vi "Sprinklernew.vi"() -> ()   [LabVIEW 2013]
doc: "This VI is the simulation of sprinkler controller.\nOn pressing Run the vi will read the data from Logdata.txt file and write it into the Zone Setup Array.\nSetup: On pressing it Zone Setup Array will enable and Zone selector allow the user to select and change the zone:\n-North\n-East\n-South\n-West\nThe controller could handle zones in any order and more than once in Zone Setup Array.\n\n In run selector toggle switch :\n-Single(off): The controller will service the Zone as setup in the zone.\n-Contineous(on):The controller will continue th ecyale as setup in zone till the Stop button will not pressed.\nStart button: It start the controller."
uses:
  Controls/Sprinkler State.ctl
  Controls/Log data states.ctl
panel:
  in  "Setup":bool
  in  "Zone Setup Array":cluster{"Zone Selector":string, "Timing":dbl}[](array[cluster])
  out "Controller Status":string
  out "Zone Indicators":T1
  in  "Water Pressure Sensor (%)":u32(slide) scale=0.0..100.0
  in  "Rain Sensor":bool
  in  "Run Selector":bool
  in  "Start":bool
  in  "stop":bool
  # "Controls"
  # "Simulation Controls"
  # "Rain"
  # "No Rain"
  # "Continuous"
  # "Single"
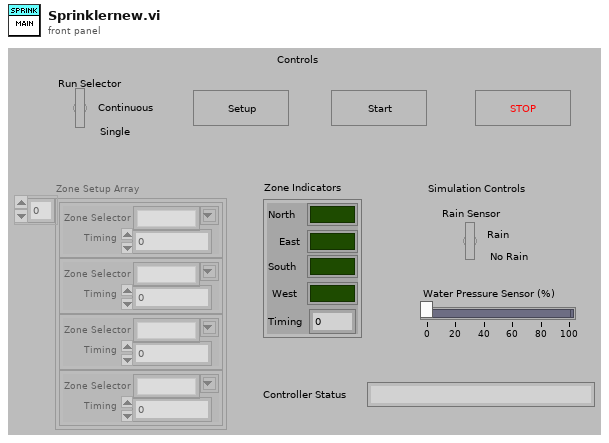
[diagram p1: front panel]
types:
  T1 = cluster{"North":bool, "East":bool, "South":bool, "West":bool, "Timing":u32}
  T2 = typedef "Sprinkler State.ctl" = enum16{"Initialize", "Setup", "Enable Zone", "Select", "Main", "Run Complete", "Rain", "Stop"}
  T3 = typedef "Log data states.ctl" = enum16{"Initialize", "Read", "Write", "Stop"}
  T4 = enum8{"Enabled", "Disabled", "Disabled and Grayed Out"}
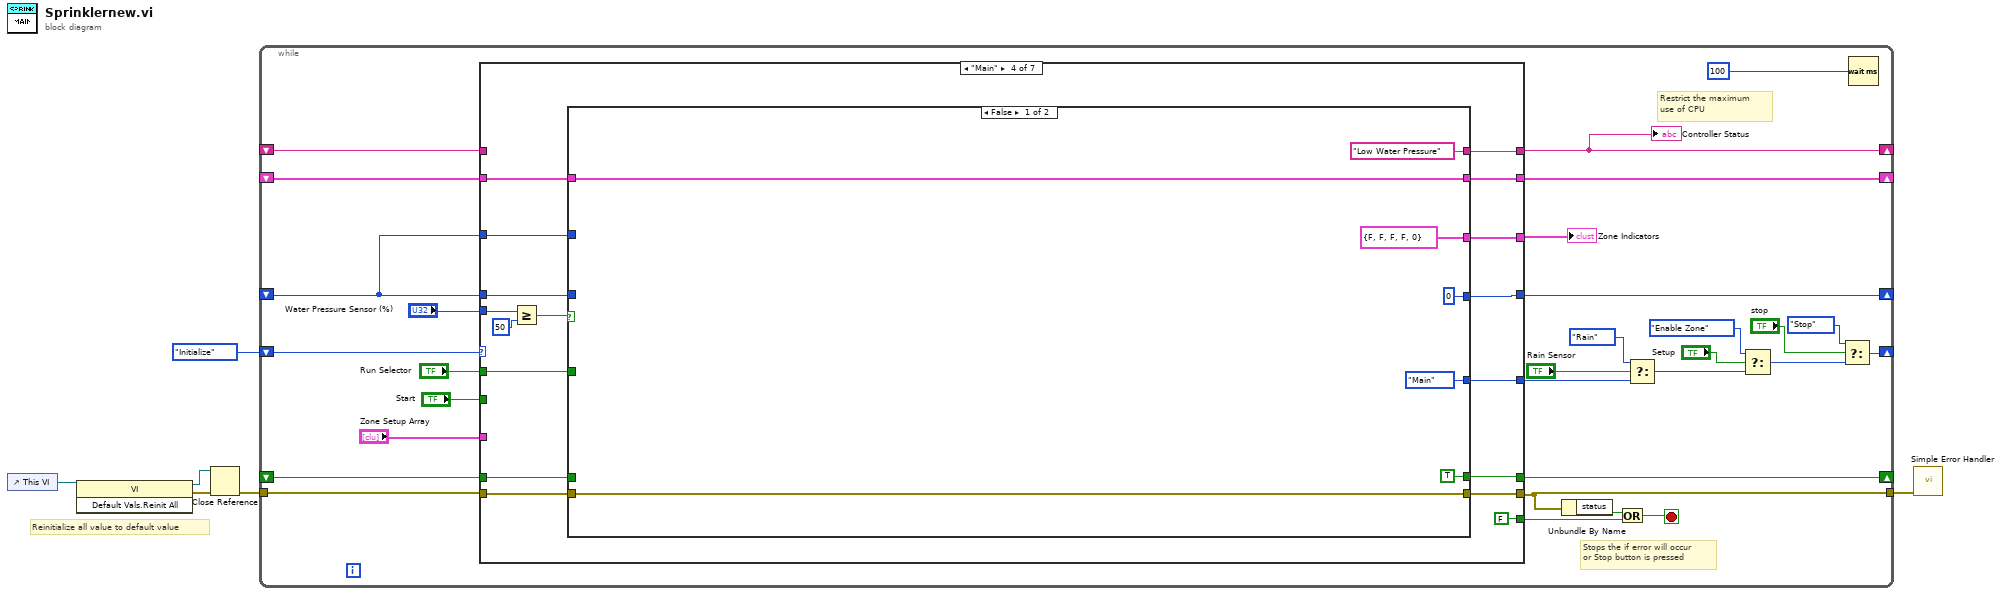
[diagram p0: block diagram]
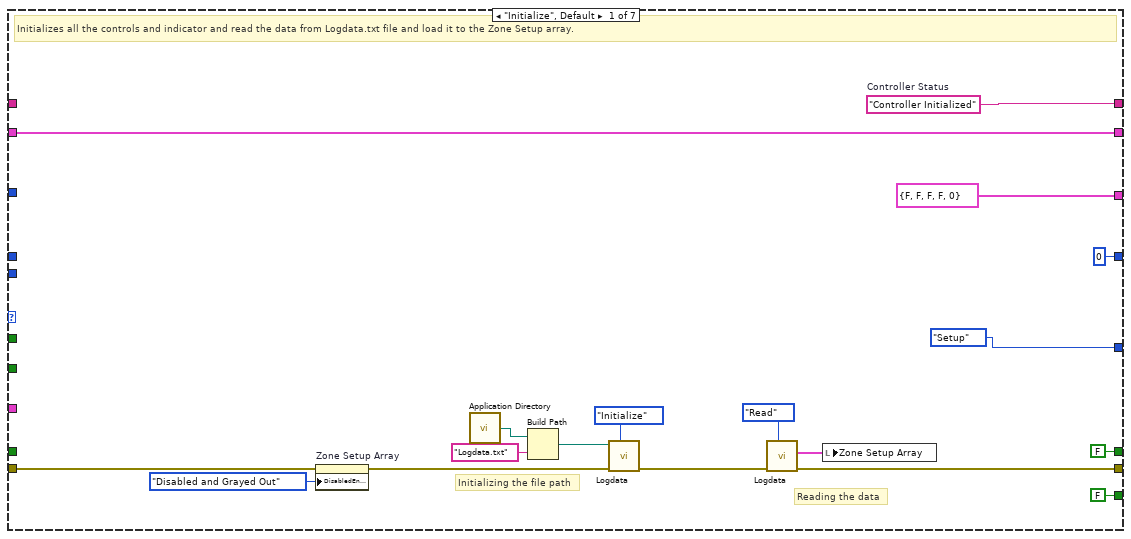
[diagram p2: hidden frame]
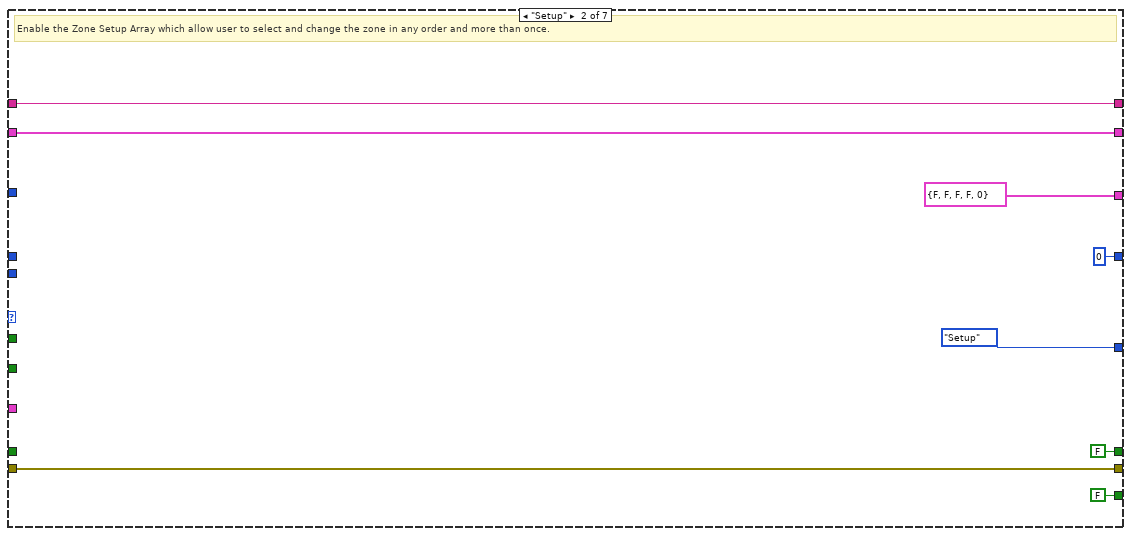
[diagram p3: hidden frame]
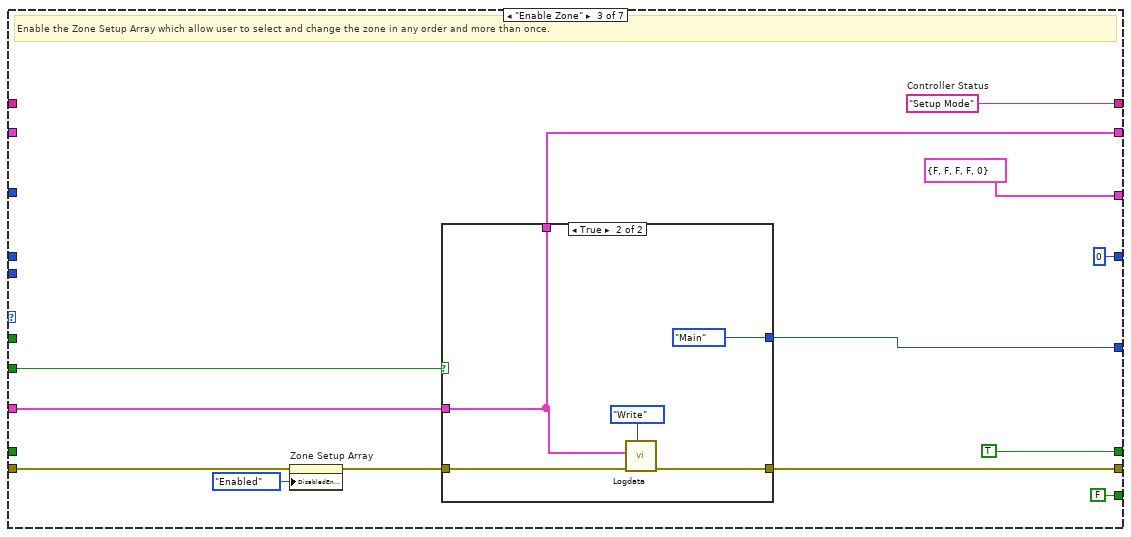
[diagram p4: hidden frame]
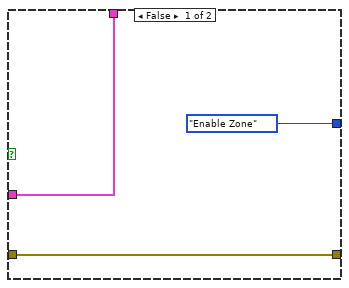
[diagram p5: hidden frame]
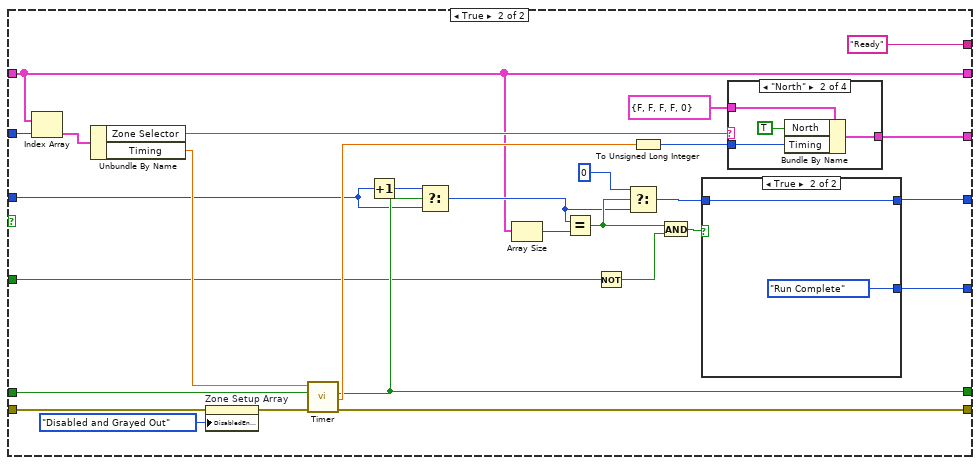
[diagram p6: hidden frame]
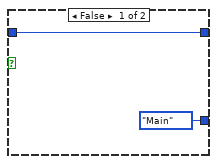
[diagram p7: hidden frame]
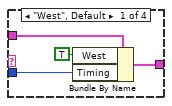
[diagram p8: hidden frame]
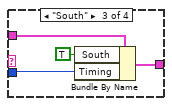
[diagram p9: hidden frame]
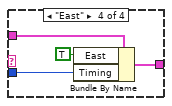
[diagram p10: hidden frame]
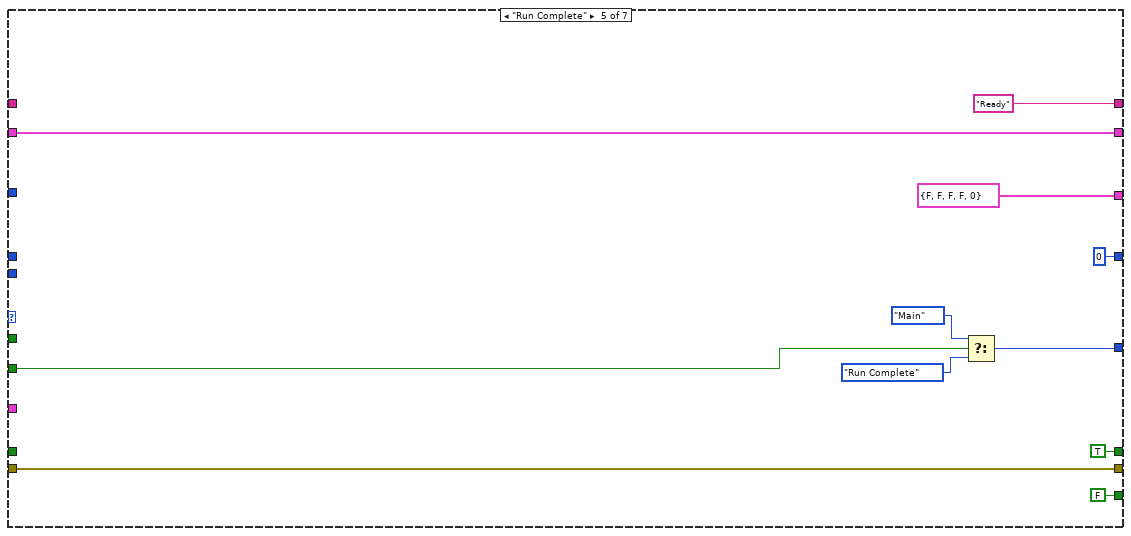
[diagram p11: hidden frame]
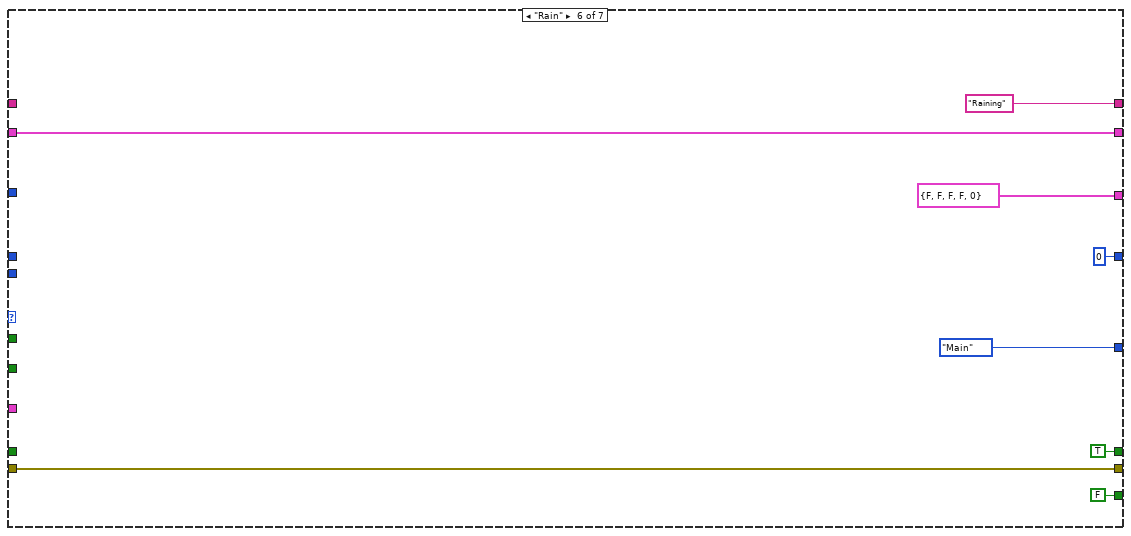
[diagram p12: hidden frame]
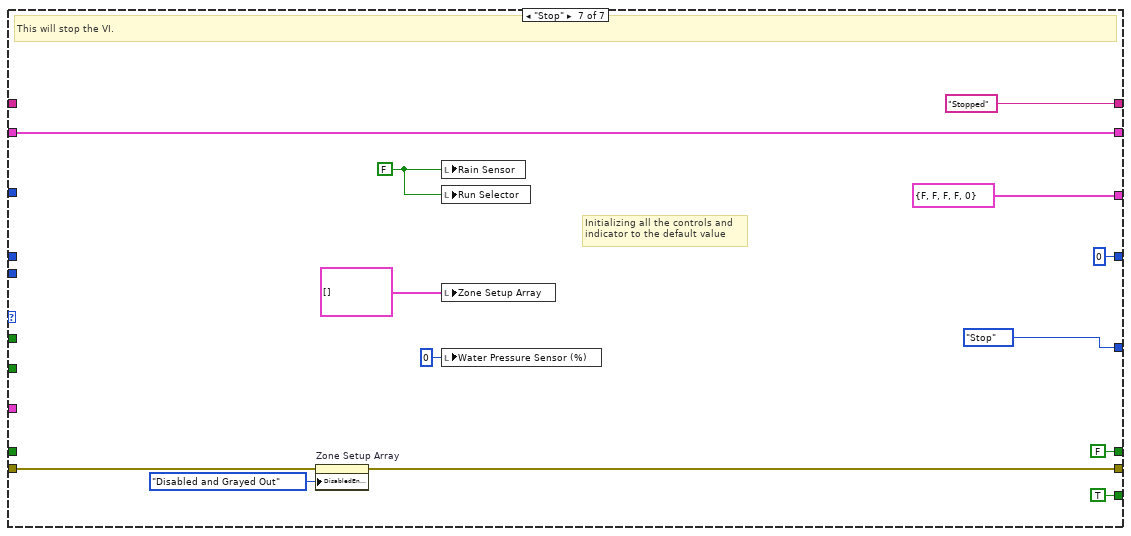
[diagram p13: hidden frame]
diagram:
  # "Reinitialize all value to default value"
  n1 = control-ref of="This VI"() -> (w6:refnum<vi>)
  n2 = invoke class="VI" method="Default Vals.Reinit All"(reference=w6) -> (reference out=w4:refnum<vi>, error out=w5:errorcluster)  [unwired: 2 in, 1 out]
  n3 = Close Reference(reference=w4, error in (no error)=w5) -> (error out=w3:errorcluster)
  n4 = while {
    tunnel: w3 -> [w35]
    tunnel: [w34] -> w2
    shift-right: [w23] -> _
    shift-left: Sprinkler_State."Initialize" -> [w30]
    shift-right: [w26] -> _
    shift-left: _ -> [w29]
    shift-right: [w18] -> _
    shift-left: _ -> [w17]
    shift-right: [w14] -> _
    shift-left: _ -> [w13]
    shift-right: [w16] -> _
    shift-left: _ -> [w15]
    stop <- w32 stop-if-true
    # "Stops the if error will occur\nor Stop button is pressed"
    # "Restrict the maximum \nuse of CPU"
    n5 = case shown="\"Main\"" w30 {
      tunnel: w35 -> [w54 w62 w64 w100 w166 w174 w187]
      tunnel: [w52 w62 w72 w95 w166 w174 w184] -> w34
      tunnel: [FALSE FALSE FALSE FALSE FALSE FALSE TRUE] -> w31
      tunnel: w29 -> [_ w61 _ _ _ _ _]
      tunnel: [w48 w61 w73 w98 "Ready" ("Controller Status") "Raining" ("Controller Status") "Stopped" ("Controller Status")] -> w26
      tunnel: "Zone Setup Array" -> [_ _ w69 _ _ _ _]
      tunnel: [T1 {"North"=FALSE, "East"=FALSE, "South"=FALSE, "West"=FALSE, "Timing"=0} ("Zone Indicators") T1 {"North"=FALSE, "East"=FALSE, "South"=FALSE, "West"=FALSE, "Timing"=0} ("Zone Indicators") T1 {"North"=FALSE, "East"=FALSE, "South"=FALSE, "West"=FALSE, "Timing"=0} ("Zone Indicators") w96 T1 {"North"=FALSE, "East"=FALSE, "South"=FALSE, "West"=FALSE, "Timing"=0} ("Zone Indicators") T1 {"North"=FALSE, "East"=FALSE, "South"=FALSE, "West"=FALSE, "Timing"=0} ("Zone Indicators") T1 {"North"=FALSE, "East"=FALSE, "South"=FALSE, "West"=FALSE, "Timing"=0} ("Zone Indicators")] -> w27
      tunnel: [Sprinkler_State."Setup" Sprinkler_State."Setup" w70 w90 w160 Sprinkler_State."Main" ("t") Sprinkler_State."Stop" ("t")] -> w11
      tunnel: "Start" -> [_ _ w71 _ w159 _ _]
      tunnel: [w45 w57 w68 w84 w163 w171 w178] -> w18
      tunnel: w17 -> [w45 w57 _ w91 w163 w171 w178]
      tunnel: w13 -> [_ _ _ w97 _ _ _]
      tunnel: [FALSE ("Elapsed?") FALSE ("Elapsed?") TRUE w93 TRUE ("Elapsed?") TRUE ("Elapsed?") FALSE ("Elapsed?")] -> w16
      tunnel: w15 -> [_ _ _ w94 _ _ _]
      tunnel: [0 0 0 w88 0 ("t") 0 ("t") 0] -> w14
      tunnel: w13 -> [_ _ _ w92 _ _ _]
      tunnel: "Run Selector" -> [_ _ _ w89 _ _ _]
      tunnel: "Water Pressure Sensor (%)" -> [_ _ _ w87 _ _ _]
      frame "Initialize", Default {
        w48 = "Controller Initialized"  # Controller Status
        # "Reading the data"
        # "Initializing the file path"
        # "Initializes all the controls and indicator and read the data from Logdata.txt file and load it to the Zone Setup array."
        n6 = property on="Zone Setup Array" class="Arr (strict)"(error in=w54, "DisabledEnum"=T4."Disabled and Grayed Out" ("Disabled")) -> (error out=w44:errorcluster)  [unwired: 1 in, 1 out]
        n7 = call <vilib>:"Application Directory.vi"() -> ("Application Directory"=w51:path)
        n8 = Build Path(base path=w51, name or relative path="Logdata.txt") -> (appended path=w39:path)
        n9 = call "Logdata.vi"("Command"=Log_data_states."Initialize", "error in (no error)"=w44, "file path (dialog if empty)"=w39) -> ("error out"=w43:errorcluster)  [unwired: 7 in, 1 out]
        n10 = call "Logdata.vi"("Command"=Log_data_states."Read", "error in (no error)"=w43) -> ("error out"=w52:errorcluster, "Zone Setup Array"=w40:cluster{"Zone Selector":string, "Timing":dbl}[])  [unwired: 8 in]
        n11 = local write "Zone Setup Array"(w40) -> ()
      }
      frame "Setup" {
        # "Enable the Zone Setup Array which allow user to select and change the zone in any order and more than once."
      }
      frame "Enable Zone" {
        w73 = "Setup Mode"  # Controller Status
        # "Enable the Zone Setup Array which allow user to select and change the zone in any order and more than once."
        n12 = property on="Zone Setup Array" class="Arr (strict)"(error in=w64, "DisabledEnum"=T4."Enabled" ("Disabled")) -> (error out=w63:errorcluster)  [unwired: 1 in, 1 out]
        n13 = case shown="True" w71 {
          tunnel: w63 -> [w77 w83]
          tunnel: [w77 w81] -> w72
          tunnel: [Sprinkler_State."Enable Zone" Sprinkler_State."Main"] -> w70
          tunnel: w69 -> [w76 w79]
          tunnel: [w76 w79] -> w68
          frame False {
          }
          frame True {
            n14 = call "Logdata.vi"("Command"=Log_data_states."Write", "error in (no error)"=w83, "Zone Setup Array"=w79) -> ("error out"=w81:errorcluster)  [unwired: 7 in, 1 out]
          }
        }
      }
      frame "Main" {
        n15 = Greater Or Equal?(x=w87, y=u32 50) -> (x >= y?=w85:bool)
        n16 = case shown="False" w85 {
          tunnel: w100 -> [w101 w135]
          tunnel: ["Low Water Pressure" ("Controller Status") "Ready" ("Controller Status")] -> w98
          tunnel: w97 -> [_ w132]
          tunnel: [T1 {"North"=FALSE, "East"=FALSE, "South"=FALSE, "West"=FALSE, "Timing"=0} ("Zone Indicators") w128] -> w96
          tunnel: [w101 w126] -> w95
          tunnel: w94 -> [_ w125]
          tunnel: [TRUE ("Elapsed?") w121] -> w93
          tunnel: w92 -> [_ w119]
          tunnel: w91 -> [w106 w108]
          tunnel: [Sprinkler_State."Main" ("t") w117] -> w90
          tunnel: w89 -> [_ w115]
          tunnel: [0 ("t") w113] -> w88
          tunnel: [w106 w108] -> w84
          frame False {
          }
          frame True {
            n17 = Index Array(array=w108, index=w132) -> (element=w131:cluster{"Zone Selector":string, "Timing":dbl})
            n18 = Unbundle By Name(w131) -> ("Zone Selector"=w130:string, "Timing"=w124:dbl)
            n19 = property on="Zone Setup Array" class="Arr (strict)"(error in=w135, "DisabledEnum"=T4."Disabled and Grayed Out" ("Disabled")) -> (error out=w127:errorcluster)  [unwired: 1 in, 1 out]
            n20 = call "Timer.vi"("error in (no error)"=w127, "Reset"=w125, "Target Time"=w124) -> ("error out"=w126:errorcluster, "Elapsed?"=w121:bool, "Elapsed TIme"=w123:dbl)  [unwired: 6 in]
            n21 = Increment(x=w119) -> (x+1=w120:i32)
            n22 = Select(t=w120, s=w121, f=w119) -> (s? t:f=w111:i32)
            n23 = Array Size(array=w108) -> (size(s)=w118:i32)
            n24 = Equal?(x=w111, y=w118) -> (x = y?=w112:bool)
            n25 = Not(x=w115) -> (.not. x?=w114:bool)
            n26 = Select(t=0, s=w112, f=w111) -> (s? t:f=w109:i32)
            n27 = To Unsigned Long Integer(number=w123) -> (unsigned 32bit integer=w122:u32)
            n28 = And(x=w112, y=w114) -> (x .and. y?=w116:bool)
            n29 = case shown="True" w116 {
              tunnel: [Sprinkler_State."Main" ("t") Sprinkler_State."Run Complete" ("t")] -> w117
              tunnel: [w136 w138] -> w113
              tunnel: w109 -> [w136 w138]
              frame False {
              }
              frame True {
              }
            }
            n30 = case shown="\"North\"" w130 {
              tunnel: T1 {"North"=FALSE, "East"=FALSE, "South"=FALSE, "West"=FALSE, "Timing"=0} ("Zone Indicators") -> [w143 w146 w150 w153]
              tunnel: [w142 w145 w149 w154] -> w128
              tunnel: w122 -> [w140 w144 w148 w152]
              frame "West", Default {
                n31 = Bundle By Name(cluster=w143, "West"=TRUE, "Timing"=w140) -> (w142:T1)
              }
              frame "North" {
                n32 = Bundle By Name(cluster=w146, "North"=TRUE ("West"), "Timing"=w144) -> (w145:T1)
              }
              frame "South" {
                n33 = Bundle By Name(cluster=w150, "South"=TRUE ("West"), "Timing"=w148) -> (w149:T1)
              }
              frame "East" {
                n34 = Bundle By Name(cluster=w153, "East"=TRUE ("West"), "Timing"=w152) -> (w154:T1)
              }
            }
          }
        }
      }
      frame "Run Complete" {
        n35 = Select(t=Sprinkler_State."Main", s=w159, f=Sprinkler_State."Run Complete" ("t")) -> (s? t:f=w160:T2)
      }
      frame "Rain" {
      }
      frame "Stop" {
        w183 = FALSE ("Rain Sensor")
        # "Initializing all the controls and \nindicator to the default value"
        # "This will stop the VI."
        n36 = property on="Zone Setup Array" class="Arr (strict)"(error in=w187, "DisabledEnum"=T4."Disabled and Grayed Out" ("Disabled")) -> (error out=w184:errorcluster)  [unwired: 1 in, 1 out]
        n37 = local write "Rain Sensor"(w183) -> ()
        n38 = local write "Run Selector"(w183) -> ()
        n39 = local write "Zone Setup Array"(cluster{"Zone Selector":string, "Timing":dbl}[] [] ("Zone Setup Array")) -> ()
        n40 = local write "Water Pressure Sensor (%)"(u32 0 ("Water Pressure Sensor (%)")) -> ()
      }
    }
    "Zone Indicators" <- w27
    "Controller Status" <- w26
    n41 = Unbundle By Name(w34) -> ("status"=w33:bool)
    n42 = Or(x=w33, y=w31) -> (x .or. y?=w32:bool)
    n43 = Select(t=Sprinkler_State."Rain", s="Rain Sensor", f=w11) -> (s? t:f=w10:T2)
    n44 = Select(t=Sprinkler_State."Enable Zone", s="Setup", f=w10) -> (s? t:f=w20:T2)
    n45 = Select(t=Sprinkler_State."Stop", s="stop", f=w20) -> (s? t:f=w23:T2)
    n46 = Wait (ms)(milliseconds to wait=u32 100) -> ()  [unwired: 1 out]
  }
  n47 = call <vilib>:"Simple Error Handler.vi"("error in (no error)"=w2) -> ()  [unwired: 4 in, 5 out]
